vi "Image Process Cal Wright 2016.vi"(4 "Path":path=path "Documents/FRC/DashboardSettings.ini") -> (0 "Settings":T1, 1 "error out":errorcluster, 2 "All User Path":path, 3 "refnum":T2)   [LabVIEW 2015]
uses:
  <vilib>/Utility/config.llb/Config Data RefNum.ctl
  <vilib>/Utility/config.llb/Read Key (Double).vi
  <vilib>/Utility/config.llb/Read Key (I32).vi
  <vilib>/Utility/config.llb/NI_LVConfig.lvlib
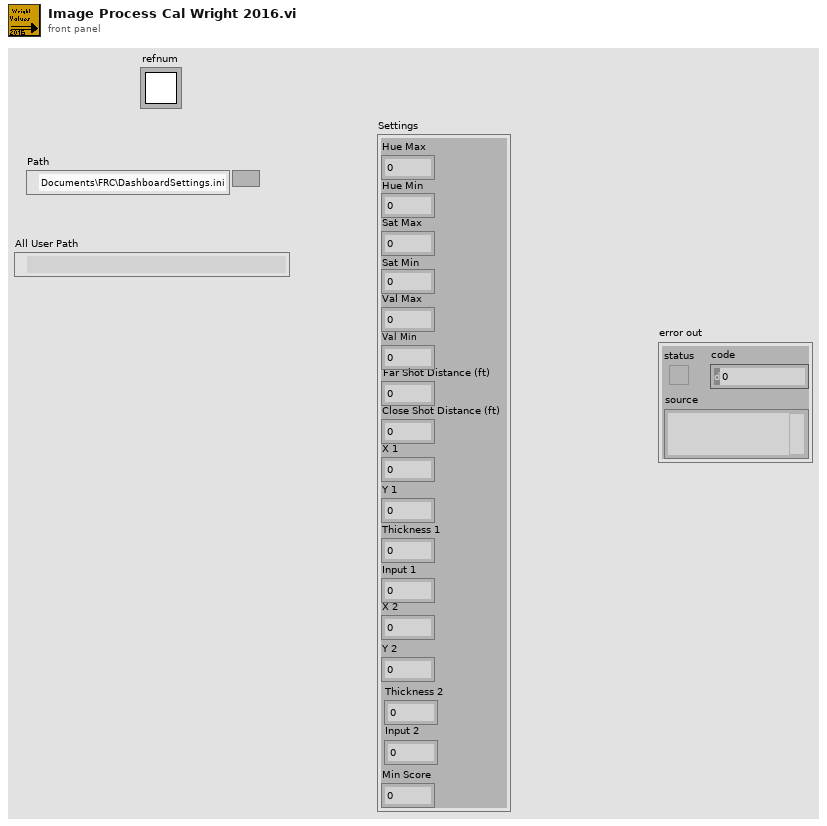
[diagram p1: front panel]
types:
  T1 = cluster{"Hue Max":dbl, "Hue Min":dbl, "Sat Max":dbl, "Sat Min":dbl, "Val Max":dbl, "Val Min":dbl, "Far Shot Distance (ft)":dbl, "Close Shot Distance (ft)":dbl, "Thickness 1":dbl, "Input 1":dbl, "X 2":dbl, "Y 2":dbl, "Thickness 2":dbl, "Input 2":dbl, "X 1":dbl, "Y 1":dbl, "Min Score":dbl}
  T2 = typedef "NI_LVConfig.lvlib/Config Data RefNum.ctl" = refnum<k1>
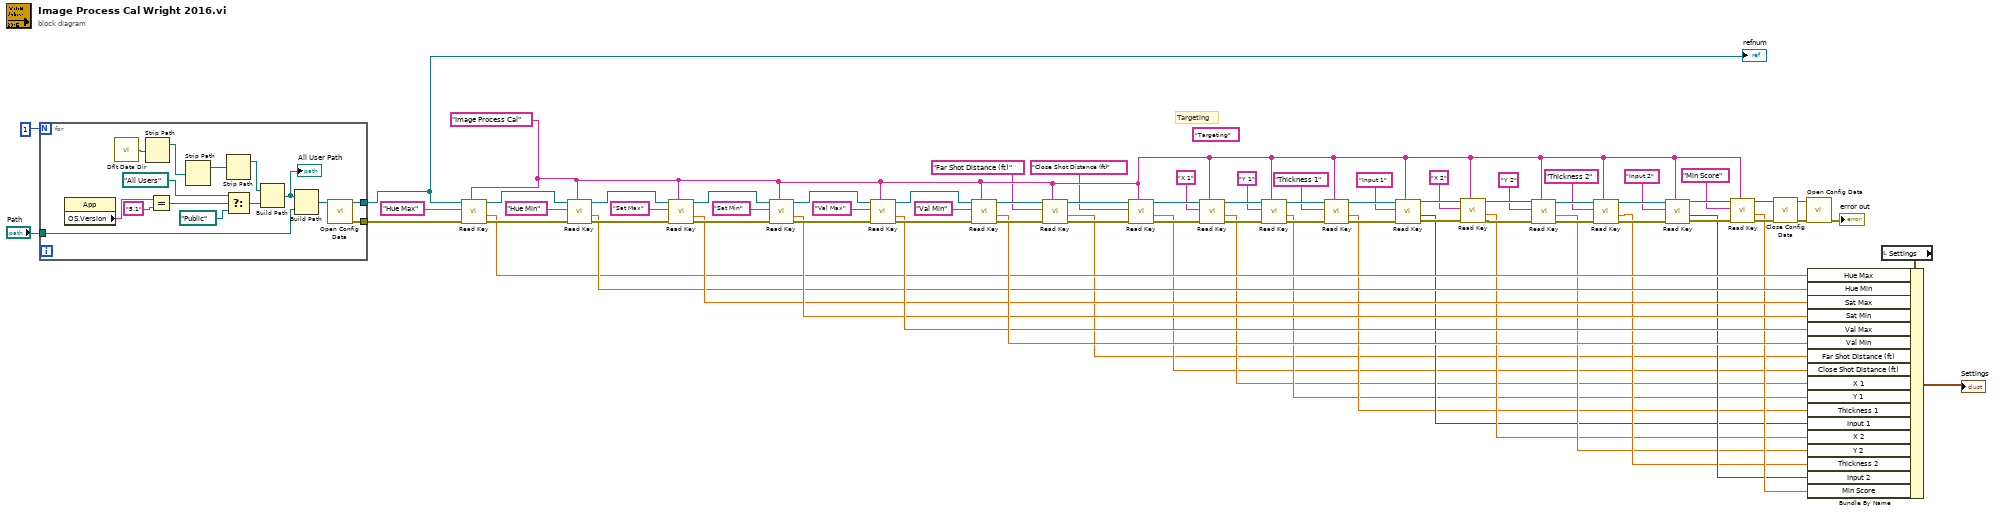
[diagram p0: block diagram]
diagram:
  (unwired) "Targeting"
  w23 = "Image Process Cal" ("section")
  # "Targeting"
  n1 = for {
    N: 1 -> [_]
    tunnel: [w81] -> w46
    tunnel: [w80] -> w45
    tunnel: "Path" -> [w79]
    n2 = property class="App"() -> ("OS.Version"=w89:string)  [unwired: 2 in, 2 out]
    n3 = call <vilib>:"Dflt Data Dir.vi"() -> ("App:Default Data Directory"=w87:path)
    n4 = Strip Path(path=w87) -> (stripped path=w88:path)  [unwired: 1 out]
    n5 = Equal?(x=w89, y="5.1") -> (x = y?=w91:bool)
    n6 = Strip Path(path=w88) -> (stripped path=w86:path)  [unwired: 1 out]
    n7 = Strip Path(path=w86) -> (stripped path=w85:path)  [unwired: 1 out]
    n8 = Select(t=path "All Users", s=w91, f=path "Public") -> (s? t:f=w84:path)
    n9 = Build Path(base path=w85, name or relative path=w84) -> (appended path=w83:path)
    "All User Path" <- w83
    n10 = Build Path(base path=w83, name or relative path=w79) -> (appended path=w82:path)
    n11 = call <vilib>:"Open Config Data.vi"("configuration file path"=w82) -> ("error out"=w81:errorcluster, "refnum"=w80:T2)  [unwired: 8 in, 1 out]
  }
  "refnum" <- w45
  n12 = call-poly <vilib>:"Read Key.vi"("section"=w23, "error in (no error)"=w46, "key"="Hue Max", "refnum"=w45) -> ("error out"=w63:errorcluster, "value"=w24:dbl, "refnum out"=w78:T2)  [unwired: 4 in, 1 out]
  n13 = call-poly <vilib>:"Read Key.vi"("section"=w23, "error in (no error)"=w63, "key"="Hue Min", "refnum"=w78) -> ("error out"=w62:errorcluster, "value"=w25:dbl, "refnum out"=w77:T2)  [unwired: 4 in, 1 out]
  n14 = call-poly <vilib>:"Read Key.vi"("section"=w23, "error in (no error)"=w62, "key"="Sat Max", "refnum"=w77) -> ("error out"=w61:errorcluster, "value"=w26:dbl, "refnum out"=w68:T2)  [unwired: 4 in, 1 out]
  n15 = call-poly <vilib>:"Read Key.vi"("section"=w23, "error in (no error)"=w61, "key"="Sat Min", "refnum"=w68) -> ("error out"=w60:errorcluster, "value"=w27:dbl, "refnum out"=w67:T2)  [unwired: 4 in, 1 out]
  n16 = call-poly <vilib>:"Read Key.vi"("section"=w23, "error in (no error)"=w60, "key"="Val Max", "refnum"=w67) -> ("error out"=w59:errorcluster, "value"=w28:dbl, "refnum out"=w75:T2)  [unwired: 4 in, 1 out]
  n17 = call-poly <vilib>:"Read Key.vi"("section"=w23, "error in (no error)"=w59, "key"="Val Min", "refnum"=w75) -> ("error out"=w58:errorcluster, "value"=w29:dbl, "refnum out"=w76:T2)  [unwired: 4 in, 1 out]
  n18 = call-poly <vilib>:"Read Key.vi"("section"=w23, "error in (no error)"=w58, "key"="Far Shot Distance (ft)", "refnum"=w76) -> ("error out"=w57:errorcluster, "value"=w1:dbl, "refnum out"=w32:T2)  [unwired: 4 in, 1 out]
  n19 = call-poly <vilib>:"Read Key.vi"("section"=w23, "error in (no error)"=w57, "key"="Close Shot Distance (ft)", "refnum"=w32) -> ("error out"=w56:errorcluster, "value"=w2:dbl, "refnum out"=w74:T2)  [unwired: 4 in, 1 out]
  n20 = call-poly <vilib>:"Read Key.vi"("section"=w23, "error in (no error)"=w56, "key"="X 1", "refnum"=w74) -> ("error out"=w55:errorcluster, "value"=w3:dbl, "refnum out"=w73:T2)  [unwired: 4 in, 1 out]
  n21 = call-poly <vilib>:"Read Key.vi"("section"=w23, "error in (no error)"=w55, "key"="Y 1", "refnum"=w73) -> ("error out"=w64:errorcluster, "value"=w4:dbl, "refnum out"=w71:T2)  [unwired: 4 in, 1 out]
  n22 = call-poly <vilib>:"Read Key.vi"("section"=w23, "error in (no error)"=w64, "key"="Thickness 1", "refnum"=w71) -> ("error out"=w65:errorcluster, "value"=w5:dbl, "refnum out"=w72:T2)  [unwired: 4 in, 1 out]
  n23 = call-poly <vilib>:"Read Key.vi"("section"=w23, "error in (no error)"=w65, "key"="Input 1", "refnum"=w72) -> ("error out"=w66:errorcluster, "value"=w6:i32, "refnum out"=w70:T2)  [unwired: 4 in, 1 out]
  n24 = call-poly <vilib>:"Read Key.vi"("section"=w23, "error in (no error)"=w66, "key"="X 2", "refnum"=w70) -> ("error out"=w35:errorcluster, "value"=w7:dbl, "refnum out"=w36:T2)  [unwired: 4 in, 1 out]
  n25 = call-poly <vilib>:"Read Key.vi"("section"=w23, "error in (no error)"=w35, "key"="Y 2", "refnum"=w36) -> ("error out"=w37:errorcluster, "value"=w8:dbl, "refnum out"=w41:T2)  [unwired: 4 in, 1 out]
  n26 = call-poly <vilib>:"Read Key.vi"("section"=w23, "error in (no error)"=w37, "key"="Thickness 2", "refnum"=w41) -> ("error out"=w38:errorcluster, "value"=w9:dbl, "refnum out"=w42:T2)  [unwired: 4 in, 1 out]
  n27 = call-poly <vilib>:"Read Key.vi"("section"=w23, "error in (no error)"=w38, "key"="Input 2", "refnum"=w42) -> ("error out"=w39:errorcluster, "value"=w10:i32, "refnum out"=w40:T2)  [unwired: 4 in, 1 out]
  n28 = call-poly <vilib>:"Read Key.vi"("section"=w23, "error in (no error)"=w39, "key"="Min Score", "refnum"=w40) -> ("error out"=w33:errorcluster, "value"=w11:dbl, "refnum out"=w34:T2)  [unwired: 4 in, 1 out]
  n29 = call <vilib>:"Close Config Data.vi"("error in (no error)"=w33, "refnum"=w34) -> ("error out"=w54:errorcluster, "file path"=w69:path)  [unwired: 1 in, 7 out]
  n30 = call <vilib>:"Open Config Data.vi"("error in (no error)"=w54, "configuration file path"=w69) -> ("error out"=→"error out":errorcluster)  [unwired: 7 in, 2 out]
  n31 = local read "Settings"() -> (w31:T1)
  n32 = Bundle By Name(cluster=w31, "Hue Max"=w24, "Hue Min"=w25, "Sat Max"=w26, "Sat Min"=w27, "Val Max"=w28, "Val Min"=w29, "Far Shot Distance (ft)"=w1, "Close Shot Distance (ft)"=w2, "X 1"=w3, "Y 1"=w4, "Thickness 1"=w5, "Input 1"=w6, "X 2"=w7, "Y 2"=w8, "Thickness 2"=w9, "Input 2"=w10, "Min Score"=w11) -> (→"Settings":T1)
